vi "ManualScan.vi"(8 "Button-OK":bool, 10 "menu reference":refnum<k9>, 11 "SN Length":string) -> (1 "MainProcess":T1=enum."TestInitialize", 3 "Barcode out:":string="6921505026477")   [LabVIEW 2013]
uses:
  Control/SystemProcess.ctl
  <vilib>/Utility/error.llb/whitespace.ctl
  Control/Buffer.vi
panel:
  in  "Button-Cancel":bool
  in  "Barcode(S/N):":string="6921505026477\n"
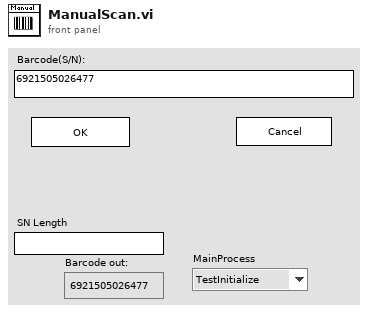
[diagram p1: front panel]
types:
  T1 = typedef "SystemProcess.ctl" = enum16{"Idle", "SystemInit", "SpecialEvent", "Barcode(SN)", "TestInitialize", "Test", "Stop", "SaveTestData", "Exit"}
  T2 = typedef "whitespace.ctl" = u16
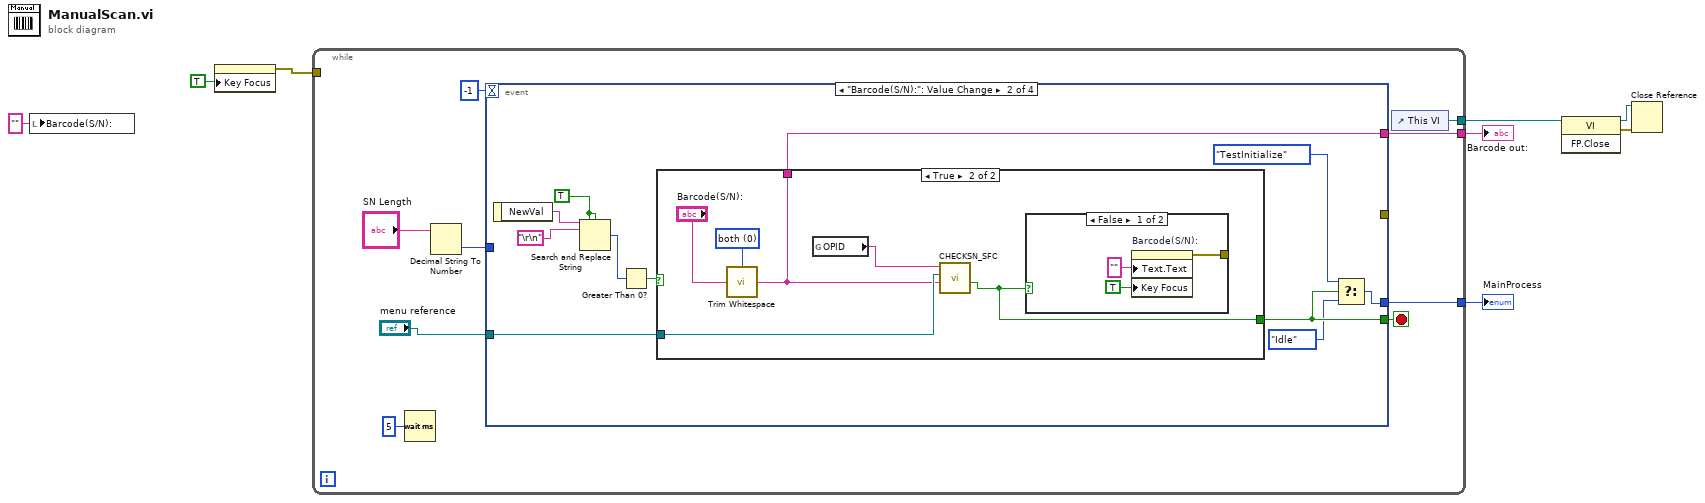
[diagram p0: block diagram]
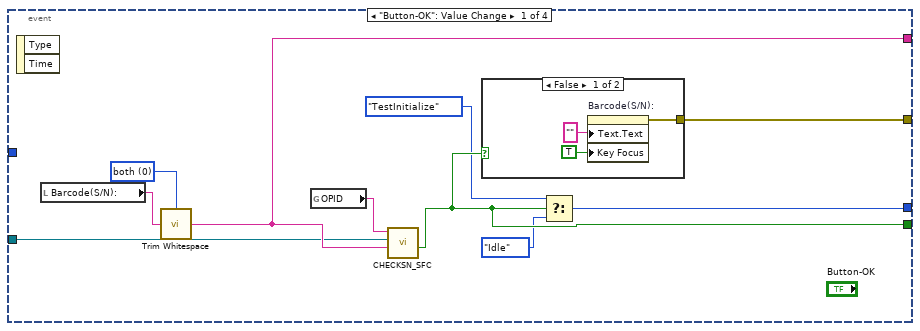
[diagram p2: hidden frame]
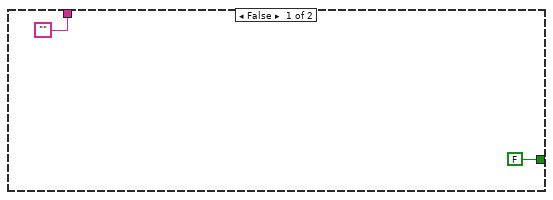
[diagram p4: hidden frame]
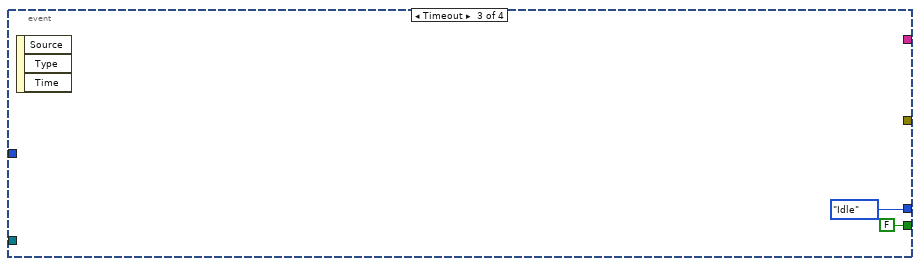
[diagram p6: hidden frame]
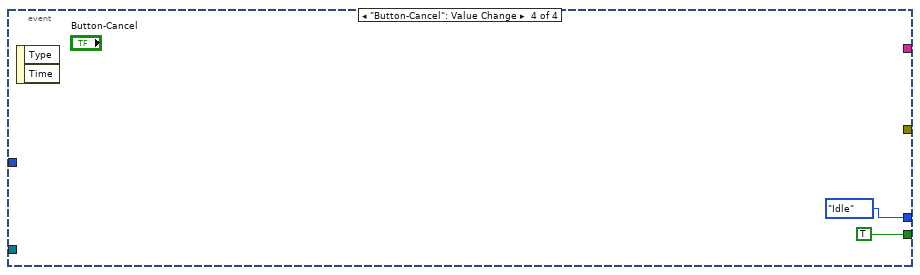
[diagram p7: hidden frame]
diagram:
  n1 = local write "Barcode(S/N):"("" ("Barcode(S/N):")) -> ()
  n2 = property on="Barcode(S/N):" class="Str"("Key Focus"=TRUE) -> (error out=w3:errorcluster)  [unwired: 2 in, 1 out]
  n3 = while {
    tunnel: [w17] -> w5
    tunnel: [w16] -> w4
    tunnel: w3 -> [_]
    tunnel: [w14] -> w2
    stop <- w15 stop-if-true
    n4 = Wait (ms)(milliseconds to wait=u32 5) -> ()  [unwired: 1 out]
    n5 = Decimal String To Number(string="SN Length") -> (number=w11:i32)  [unwired: 2 in, 1 out]
    n6 = event shown="[1] \"Barcode(S/N):\": Value Change" {
      selector: _ -> [_ _ _ _]
      dyn-events: _ -> [_ _ _ _]
      timeout: -1 -> [_ _ _ _]
      tunnel: [w26 w39 FALSE ("OK in") TRUE ("OK in")] -> w15
      tunnel: [w24 w41 _ _] -> w16
      tunnel: [w27 w37 SystemProcess."Idle" ("MainProcess") SystemProcess."Idle" ("MainProcess")] -> w14
      tunnel: [w25 _ _ _] -> _
      tunnel: w11 -> [_ _ _ _]
      tunnel: "menu reference" -> [w18 w40 _ _]
      event "Button-OK": Value Change {
        w19 = T2 0 items=["both", "start of string", "end of string"] ("location (both)")
        n7 = event-data() -> ()  [unwired: 1 in, 2 out]
        n8 = local read "Barcode(S/N):"() -> (w20:string)
        n9 = call <vilib>:"Trim Whitespace.vi"("string"=w20, "location (both)"=w19) -> ("trimmed string"=w24:string)
        n10 = global read "Buffer.vi" "OPID"() -> (w21:string)
        n11 = call "CHECKSN_SFC.vi"("SN"=w24, "menu reference"=w18, "OPID"=w21) -> ("SNCheck"=w26:bool)  [unwired: 7 in, 1 out]
        n12 = case shown="False" w26 {
          tunnel: [w28 _] -> w25
          frame False {
            n13 = property on="Barcode(S/N):" class="Str"("Text.Text"="", "Key Focus"=TRUE) -> (error out=w28:errorcluster)  [unwired: 2 in, 1 out]
          }
          frame True {
          }
        }
        n14 = Select(t=SystemProcess."TestInitialize" ("MainProcess"), s=w26, f=SystemProcess."Idle") -> (s? t:f=w27:T1)
      }
      event "Barcode(S/N):": Value Change {
        w34 = TRUE ("replace all? (F)")
        n15 = event-data() -> ("NewVal"=w35:string)  [unwired: 1 in]
        n16 = Search and Replace String(replace all?=w34, case sensitive?=w34, input string=w35, search string="\r\n") -> (number of replacements=w31:i32)  [unwired: 4 in, 3 out]
        n17 = Greater Than 0?(x=w31) -> (x > 0?=w32:bool)
        n18 = case shown="True" w32 {
          tunnel: ["" w45] -> w41
          tunnel: [FALSE w47] -> w39
          tunnel: w40 -> [_ w46]
          frame False {
          }
          frame True {
            w44 = T2 0 items=["both", "start of string", "end of string"] ("location (both)")
            n19 = call <vilib>:"Trim Whitespace.vi"("string"="Barcode(S/N):", "location (both)"=w44) -> ("trimmed string"=w45:string)
            n20 = global read "Buffer.vi" "OPID"() -> (w49:string)
            n21 = call "CHECKSN_SFC.vi"("SN"=w45, "menu reference"=w46, "OPID"=w49) -> ("SNCheck"=w47:bool)  [unwired: 7 in, 1 out]
            n22 = case shown="False" w47 {
              tunnel: [w50 _] -> _
              frame False {
                n23 = property on="Barcode(S/N):" class="Str"("Text.Text"="", "Key Focus"=TRUE) -> (error out=w50:errorcluster)  [unwired: 2 in, 1 out]
              }
              frame True {
              }
            }
          }
        }
        n24 = Select(t=SystemProcess."TestInitialize" ("MainProcess"), s=w39, f=SystemProcess."Idle" ("MainProcess")) -> (s? t:f=w37:T1)
      }
      event Timeout {
        n25 = event-data() -> ()  [unwired: 1 in, 3 out]
      }
      event "Button-Cancel": Value Change {
        n26 = event-data() -> ()  [unwired: 1 in, 2 out]
      }
    }
    n27 = control-ref of="This VI"() -> (w17:refnum<vi>)
  }
  "Barcode out:" <- w4
  "MainProcess" <- w2
  n28 = invoke class="VI" method="FP.Close"(reference=w5) -> (reference out=w7:refnum<vi>, error out=w6:errorcluster)  [unwired: 2 in, 1 out]
  n29 = Close Reference(reference=w7, error in (no error)=w6) -> ()  [unwired: 1 out]
